vi "String aufbereiten.vi"(5 "read buffer":string) -> (6 "String":string)   [LabVIEW 2020, in "AK-Schnittstelle.lvlib"]
uses:
  AK-Schnittstelle.lvlib
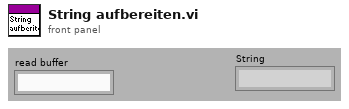
[diagram p1: front panel]
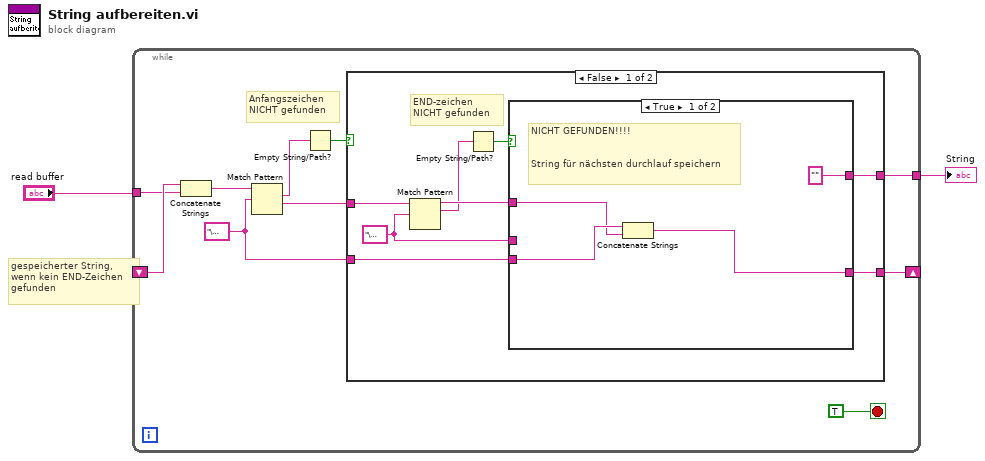
[diagram p0: block diagram]
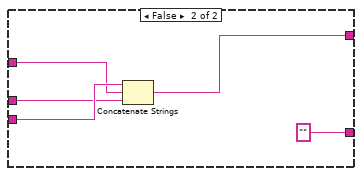
[diagram p2: hidden frame]
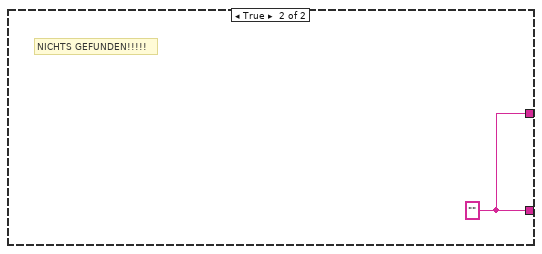
[diagram p3: hidden frame]
diagram:
  # "gespeicherter String,\nwenn kein END-Zeichen\ngefunden"
  n1 = while {
    shift-right: [w9] -> _
    shift-left: _ -> [w8]
    tunnel: "read buffer" -> [w7]
    tunnel: [w5] -> w1
    stop <- TRUE stop-if-true
    w11 = "\u0002" ("String")
    # "Anfangszeichen \nNICHT gefunden"
    n2 = Concatenate Strings(w8, w7) -> (w6:string)
    n3 = Match Pattern(string=w6, regular expression=w11) -> (match substring=w3:string, after substring=w12:string)  [unwired: 1 in, 2 out]
    n4 = Empty String/Path?(string/path=w3) -> (empty?=w4:bool)
    n5 = case shown="False" w4 {
      tunnel: [w20 w30] -> w5
      tunnel: w12 -> [w19 _]
      tunnel: w11 -> [w17 _]
      tunnel: [w16 w30] -> w9
      frame False {
        w13 = "\u0003" ("String")
        # "END-zeichen \nNICHT gefunden"
        n6 = Match Pattern(string=w19, regular expression=w13) -> (before substring=w18:string, match substring=w15:string)  [unwired: 1 in, 2 out]
        n7 = Empty String/Path?(string/path=w15) -> (empty?=w14:bool)
        n8 = case shown="True" w14 {
          tunnel: ["" ("read buffer") w25] -> w20
          tunnel: w18 -> [w23 w28]
          tunnel: w17 -> [w24 w29]
          tunnel: [w22 "" ("read buffer")] -> w16
          tunnel: w13 -> [_ w26]
          frame True {
            # "NICHT GEFUNDEN!!!!\n\n\nString für nächsten durchlauf speichern"
            n9 = Concatenate Strings(w24, w23) -> (w22:string)
          }
          frame False {
            n10 = Concatenate Strings(w29, w28, w26) -> (w25:string)
          }
        }
      }
      frame True {
        w30 = ""
        # "NICHTS GEFUNDEN!!!!!"
      }
    }
  }
  "String" <- w1
